vi "DoNanoOpSendCmdRcvResp.vi"(7 "Expected response time (msecs)":u32=3000, 8 "error in (no error)":errorcluster, 9 "Wait after response":bool=TRUE, 10 "Cmd String":string, 11 "VISA resource name":refnum<visa-resource-name>) -> (0 "error out":errorcluster, 1 "Line 2":string, 2 "Line 1":string, 3 "VISA resource name out":refnum<visa-resource-name>, 4 "Line 4":string, 5 "Line 3":string, 6 "read buffer":string)   [LabVIEW 2013]
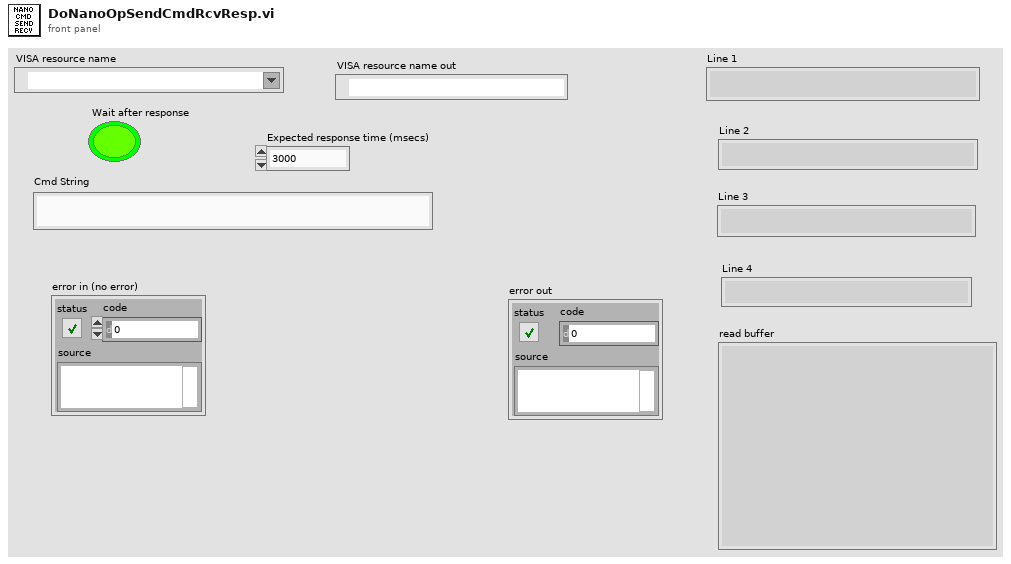
[diagram p1: front panel]
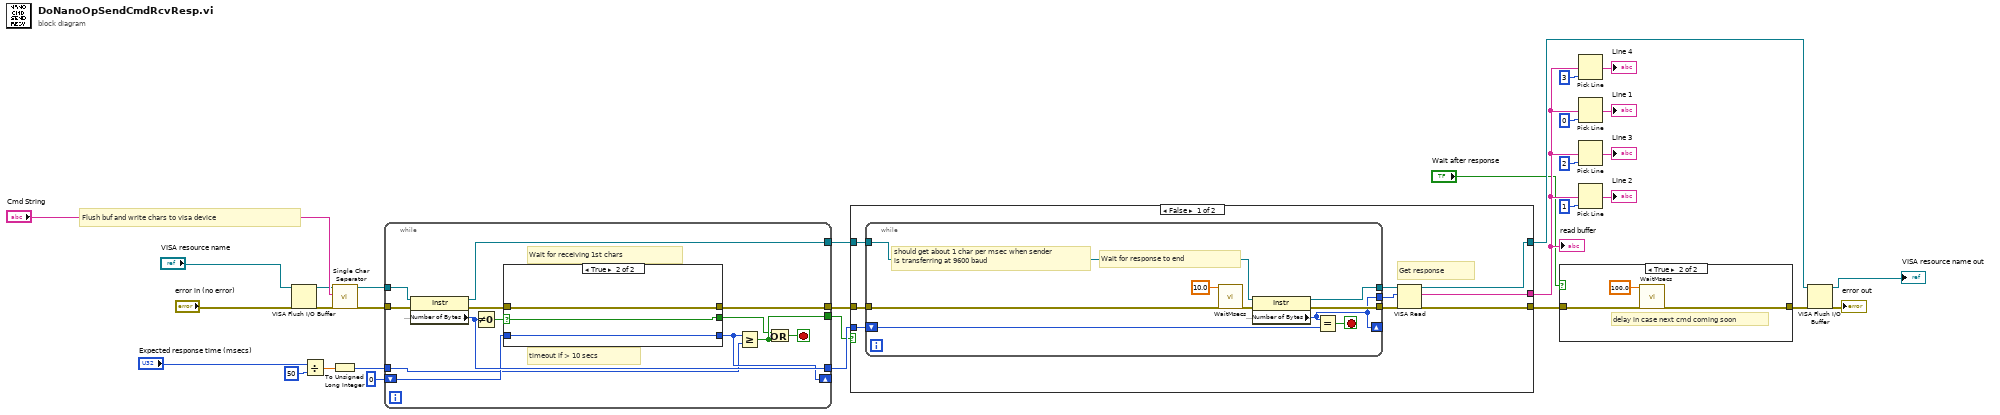
[diagram p0: block diagram]
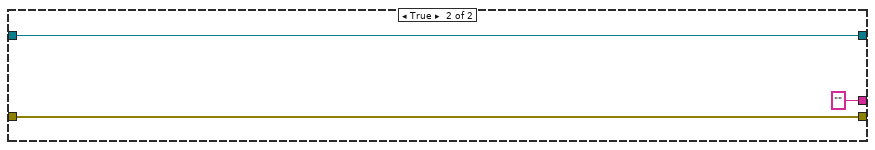
[diagram p2: hidden frame]
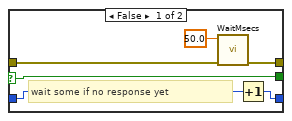
[diagram p3: hidden frame]
diagram:
  # "Flush buf and write chars to visa device"
  n1 = VISA Flush I/O Buffer(VISA resource name="VISA resource name", error in (no error)="error in (no error)") -> (VISA resource name out=w8:refnum<visa-resource-name>, error out=w9:errorcluster)  [unwired: 1 in]
  n2 = Divide(x="Expected response time (msecs)", y=u32 50) -> (x/y=w12:dbl)
  n3 = To Unsigned Long Integer(number=w12) -> (unsigned 32bit integer=w11:u32)
  n4 = call "Single Char Seperator.vi"("error in (no error)"=w9, "String"="Cmd String", "VISA resource name"=w8) -> ("error out"=w6:errorcluster, "VISA resource name 2"=w7:refnum<visa-resource-name>)  [unwired: 7 in]
  n5 = while {
    tunnel: [w32] -> w4
    tunnel: [w41] -> w3
    tunnel: [w44] -> w2
    tunnel: w7 -> [w43]
    tunnel: w6 -> [w42]
    shift-right: [w37] -> _
    shift-left: 0 -> [w40]
    tunnel: [w36] -> w1
    tunnel: w11 -> [w35]
    stop <- w38 stop-if-true
    # "Wait for receiving 1st chars"
    # "timeout if > 10 secs"
    n6 = property class="Instr"(reference=w43, error in=w42) -> (reference out=w44:refnum<visa-resource-name>, error out=w33:errorcluster, "Serial Settings:Number of Bytes at Serial Port"=w41:u32)
    n7 = Not Equal To 0?(x=w41) -> (x != 0?=w39:bool)
    n8 = case shown="True" w39 {
      selector: w39 -> [w47 w52]
      tunnel: w40 -> [w49 w53]
      tunnel: [w48 w53] -> w37
      tunnel: [w47 w52] -> w34
      tunnel: w33 -> [w46 w51]
      tunnel: [w45 w51] -> w32
      frame False {
        # "wait some if no response yet"
        n9 = call "WaitMsecs.vi"("error in (no error)"=w46, "Wait Msecs"=50.0) -> ("error out"=w45:errorcluster)  [unwired: 9 in]
        n10 = Increment(x=w49) -> (x+1=w48:i32)
      }
      frame True {
      }
    }
    n11 = Greater Or Equal?(x=w37, y=w35) -> (x >= y?=w36:bool)
    n12 = Or(x=w34, y=w36) -> (x .or. y?=w38:bool)
  }
  n13 = case shown="False" w1 {
    tunnel: [w62 w74] -> w19
    tunnel: [w61 w73] -> w17
    tunnel: [w60 "" ("read buffer")] -> w20
    tunnel: w4 -> [w59 w74]
    tunnel: w3 -> [w58 _]
    tunnel: w2 -> [w57 w73]
    frame False {
      # "Get response"
      n14 = while {
        tunnel: w59 -> [w69]
        shift-right: [w63] -> _
        shift-left: w58 -> [w68]
        tunnel: w57 -> [w66]
        tunnel: [w65] -> w56
        tunnel: [w64] -> w55
        tunnel: [w63] -> w54
        stop <- w67 stop-if-true
        # "should get about 1 char per msec when sender\nis transferring at 9600 baud"
        # "Wait for response to end"
        n15 = call "WaitMsecs.vi"("error in (no error)"=w69, "Wait Msecs"=10.0) -> ("error out"=w70:errorcluster)  [unwired: 9 in]
        n16 = property class="Instr"(reference=w66, error in=w70) -> (reference out=w65:refnum<visa-resource-name>, error out=w64:errorcluster, "Serial Settings:Number of Bytes at Serial Port"=w63:u32)
        n17 = Equal?(x=w63, y=w68) -> (x = y?=w67:bool)
      }
      n18 = VISA Read(VISA resource name=w56, byte count=w54, error in (no error)=w55) -> (VISA resource name out=w61:refnum<visa-resource-name>, read buffer=w60:string, error out=w62:errorcluster)  [unwired: 1 out]
    }
    frame True {
    }
  }
  "read buffer" <- w20
  n19 = case shown="True" "Wait after response" {
    tunnel: w19 -> [w75 w77]
    tunnel: [w75 w76] -> w18
    frame False {
    }
    frame True {
      # "delay in case next cmd coming soon"
      n20 = call "WaitMsecs.vi"("error in (no error)"=w77, "Wait Msecs"=100.0) -> ("error out"=w76:errorcluster)  [unwired: 9 in]
    }
  }
  n21 = Pick Line(multi-line string=w20, line index=3) -> (output string=→"Line 4":string)  [unwired: 1 in]
  n22 = Pick Line(multi-line string=w20, line index=0) -> (output string=→"Line 1":string)  [unwired: 1 in]
  n23 = Pick Line(multi-line string=w20, line index=2) -> (output string=→"Line 3":string)  [unwired: 1 in]
  n24 = Pick Line(multi-line string=w20, line index=1) -> (output string=→"Line 2":string)  [unwired: 1 in]
  n25 = VISA Flush I/O Buffer(VISA resource name=w17, error in (no error)=w18) -> (VISA resource name out=→"VISA resource name out":refnum<visa-resource-name>, error out=→"error out":errorcluster)  [unwired: 1 in]
